vi "Log Critical.vi"(8 "error in (no error)":errorcluster, 10 "Message":string, 11 "Logging In":refnum<class "Logging.lvclass">) -> (0 "error out":errorcluster, 3 "Logging Out":refnum<class "Logging.lvclass">)   [LabVIEW 2020, in "Logging.lvclass"]
doc: "Enter a critical-level message into the system log.\nA critical error is a serious error, indicating that the program itself may be unable to continue running.\nLogging is not meant as a substitute for error handling."
uses:
  Logging.lvclass
  Protected/Level.ctl
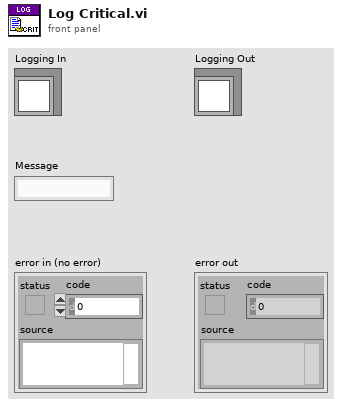
[diagram p1: front panel]
types:
  T1 = typedef "Logging.lvclass/Level.ctl" = enum16{"DEBUG", "INFO", "WARNING", "ERROR", "CRITICAL"}
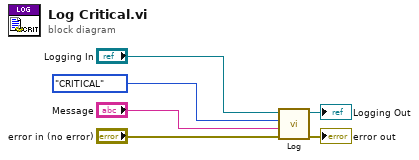
[diagram p0: block diagram]
diagram:
  n1 = call-dynamic "Log.vi"("error in (no error)"="error in (no error)", "Message"="Message", "Level"=Level."CRITICAL", "Logging In"="Logging In") -> ("error out"=→"error out":errorcluster, "Logging Out"=→"Logging Out":refnum<class "Logging.lvclass">)  [unwired: 6 in]
